vi "Send Start.vi"(8 "error in (no error)":errorcluster, 11 "Dispatcher Interface in":refnum<class "Dispatcher Interface.lvclass">) -> (0 "error out":errorcluster, 3 "Dispatcher Interface out":refnum<class "Dispatcher Interface.lvclass">)   [LabVIEW 2020, in "DSF Core.lvlib" / "Dispatcher Interface.lvclass"]
uses:
  Dispatcher Interface.lvclass
  Command.ctl
  Parameters.ctl
  Command Data.ctl
  Write Dispatcher Command.vi
  Interface.lvclass
  Response.ctl
  Read Dispatcher Response.vi
  Invalid Response.vi
  C:/Users/nitest/Desktop/Git/niveristand-data-sharing-framework-custom-device/Source/Core/Classes/Interface/Interface.lvclass
  C:/Users/nitest/Desktop/Git/niveristand-data-sharing-framework-custom-device/Source/Core/Classes/Interface/Dispatcher/Dispatcher Interface.lvclass
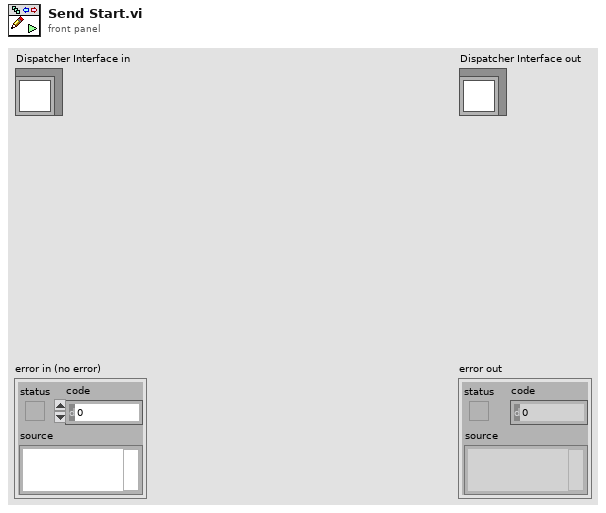
[diagram p1: front panel]
types:
  T1 = typedef "DSF Core.lvlib/Dispatcher Interface.lvclass/Command.ctl" = enum8{"Idle", "Start", "Rx", "Tx", "Set Inline Buffer", "Shutdown", "Error"}
  T2 = typedef "DSF Core.lvlib/Dispatcher Interface.lvclass/Command Data.ctl" = cluster{"Command":T1, "Parameters":T3}
  T3 = typedef "DSF Core.lvlib/Dispatcher Interface.lvclass/Parameters.ctl" = cluster{"arg1":u64, "arg2":u64}
  T4 = typedef "DSF Core.lvlib/Dispatcher Interface.lvclass/Response Data.ctl" = cluster{"Response":T5, "Parameters":T3}
  T5 = typedef "DSF Core.lvlib/Dispatcher Interface.lvclass/Response.ctl" = enum8{"General Ack", "Error", "Shutting Down"}
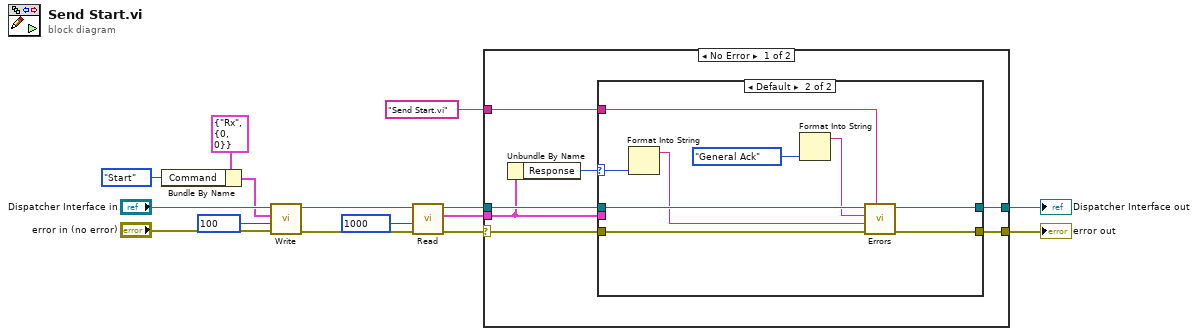
[diagram p0: block diagram]
diagram:
  n1 = Bundle By Name(cluster=T2 {"Command"=enum."Rx", "Parameters"={"arg1"=0, "arg2"=0}} ("command"), "Command"=Command."Start") -> (w11:T2)
  n2 = call-poly "Write.vi"("error in (no error)"="error in (no error)", "timeout in ms (0)"=100, "command"=w11, "Dispatcher Interface in"="Dispatcher Interface in") -> ("error out"=w4:errorcluster, "Dispatcher Interface out"=w3:refnum<class "Dispatcher Interface.lvclass">)  [unwired: 6 in]
  n3 = call-poly "Read.vi"("error in (no error)"=w4, "timeout in ms (0)"=1000, "Dispatcher Interface in"=w3) -> ("error out"=w6:errorcluster, "response"=w7:T4, "Dispatcher Interface out"=w9:refnum<class "Dispatcher Interface.lvclass">)  [unwired: 5 in, 1 out]
  n4 = case shown="No Error" w6 {
    selector: w6 -> [w17 w34]
    tunnel: [w21 w34] -> w2
    tunnel: w9 -> [w20 w35]
    tunnel: [w19 w35] -> w1
    tunnel: w7 -> [w18 _]
    tunnel: "Send Start.vi" ("error source vi name") -> [w16 _]
    frame No Error {
      n5 = Unbundle By Name(w18) -> ("Response"=w22:T5)
      n6 = case shown="Default" w22 {
        selector: w22 -> [_ w28]
        tunnel: w17 -> [w23 w32]
        tunnel: [w23 w30] -> w21
        tunnel: w20 -> [w24 w33]
        tunnel: [w24 w31] -> w19
        tunnel: w18 -> [_ _]
        tunnel: w16 -> [_ w29]
        frame "General Ack" {
        }
        frame Default {
          n7 = Format Into String(w28) -> (resulting string=w27:string)  [unwired: 3 in, 1 out]
          n8 = Format Into String(Response."General Ack" ("expected response")) -> (resulting string=w25:string)  [unwired: 3 in, 1 out]
          n9 = call-poly "Errors.vi"("error source vi name"=w29, "error in (no error)"=w32, "actual response"=w27, "expected response"=w25, "Interface in"=w33) -> ("error out"=w30:errorcluster, "Interface out"=w31:refnum<class "Dispatcher Interface.lvclass">)  [unwired: 5 in]
        }
      }
    }
    frame Error {
      # "Incoming error. Pass through."
    }
  }
  "error out" <- w2
  "Dispatcher Interface out" <- w1
